vi "GetObjects.vi"(8 "error in":errorcluster, 11 "Diagram in":refnum<class "Diagram.lvclass">) -> (0 "error out":errorcluster, 3 "Diagram out":refnum<class "Diagram.lvclass">)   [LabVIEW 2014, in "Raspberry Pi Compatible Compiler for LabVIEW.lvlib" / "Diagram.lvclass"]
uses:
  Diagram.lvclass
  Diagram.lvclass/Diagram.ctl
  Constant/Constant.lvclass
  Function/Function.lvclass
  Structure/Structure.lvclass
  GrowableFunction/GrowableFunction.lvclass
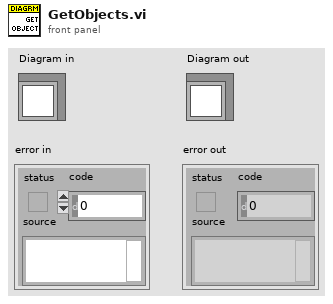
[diagram p1: front panel]
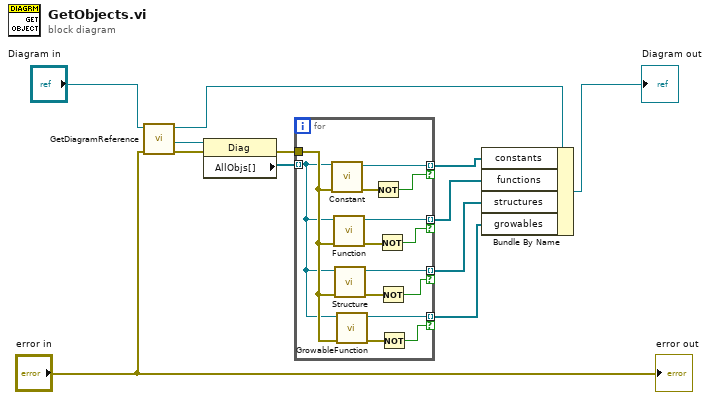
[diagram p0: block diagram]
diagram:
  n1 = call "GetDiagramReference.vi"("error in"="error in", "Diagram in"="Diagram in") -> ("error out"=w5:errorcluster, "reference out"=w4:refnum<vi>, "Diagram out"=w3:refnum<class "Diagram.lvclass">)  [unwired: 5 in]
  n2 = property class="Diag"(reference=w4, error in=w5) -> (error out=w9:errorcluster, "AllObjs[]"=w12:refnum<vi>[])  [unwired: 1 out]
  n3 = for {
    tunnel: w12 -> [w16] mode=indexing
    tunnel: [w26] -> w11 mode=indexing if=w24
    tunnel: w9 -> [w17]
    tunnel: [w22] -> w8 mode=indexing if=w21
    tunnel: [w19] -> w7 mode=indexing if=w18
    tunnel: [w15] -> w6 mode=indexing if=w13
    n4 = call "Constant.vi"("error in"=w17, "reference"=w16) -> ("error out"=w25:errorcluster, "constant out"=w26:refnum<class "Constant.lvclass">)  [unwired: 8 in]
    n5 = call "Function.vi"("error in"=w17, "reference"=w16) -> ("error out"=w23:errorcluster, "Function out"=w22:refnum<class "Function.lvclass">)  [unwired: 8 in]
    n6 = call "Structure.vi"("error in"=w17, "reference"=w16) -> ("error out"=w20:errorcluster, "structure out"=w19:refnum<class "Structure.lvclass">)  [unwired: 8 in]
    n7 = call "GrowableFunction.vi"("error in"=w17, "reference"=w16) -> ("error out"=w14:errorcluster, "Function out"=w15:refnum<class "GrowableFunction.lvclass">)  [unwired: 8 in]
    n8 = Not(x=w25) -> (.not. x?=w24:bool)
    n9 = Not(x=w23) -> (.not. x?=w21:bool)
    n10 = Not(x=w20) -> (.not. x?=w18:bool)
    n11 = Not(x=w14) -> (.not. x?=w13:bool)
  }
  n12 = Bundle By Name(cluster=w3, "constants"=w11, "functions"=w8, "structures"=w7, "growables"=w6) -> (→"Diagram out":refnum<class "Diagram.lvclass">)
  "error out" <- "error in"
